vi "build_rid_iterating.vi"(7 "ext":string="_data.h5", 8 "error in (no error)":errorcluster, 9 "save?":bool, 10 "time stamp":timestamp, 11 "base":path[](array[path])) -> (0 "error out":errorcluster, 2 "run ID":string="20180125_155324", 3 "output":path[](array[path]))   [LabVIEW 2017, in "tools.lvlib"]
uses:
  tools.lvlib
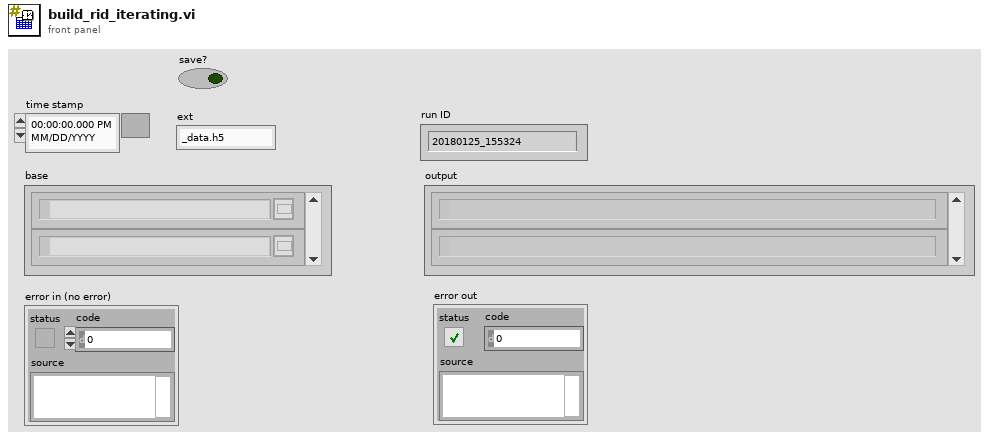
[diagram p1: front panel]
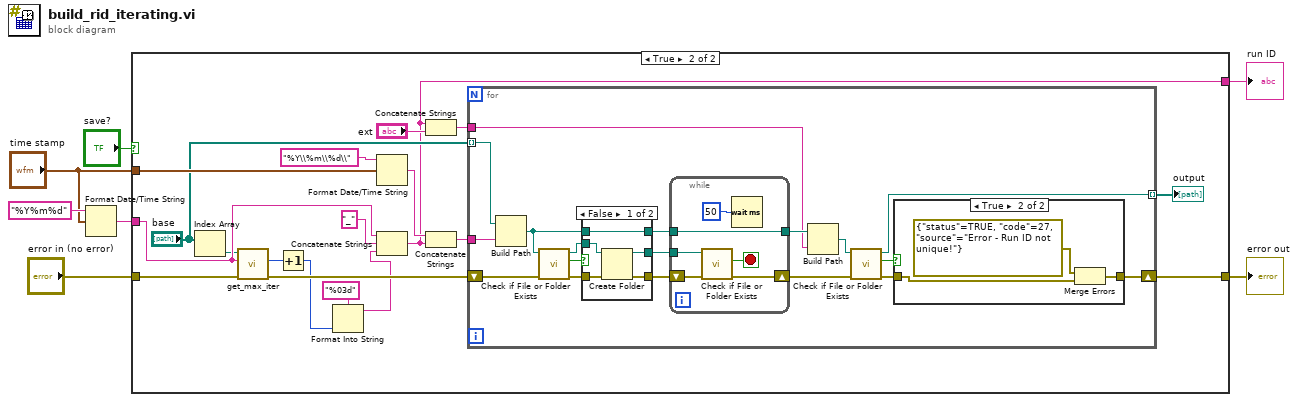
[diagram p0: block diagram]
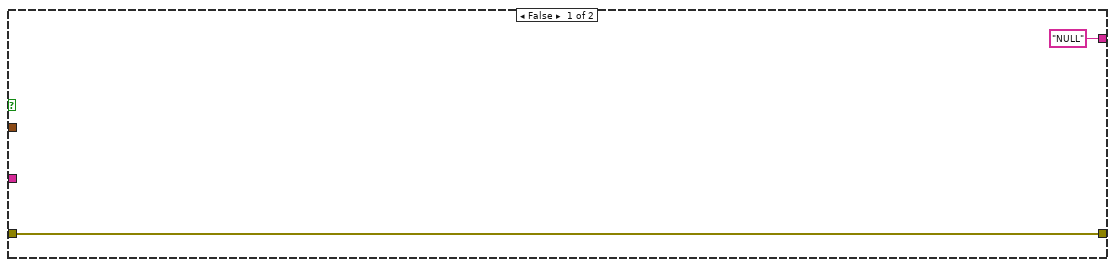
[diagram p2: hidden frame]
diagram:
  n1 = Format Date/Time String(time format string (%c)="%Y%m%d", seconds (now)="time stamp") -> (date/time string=w1:string)  [unwired: 1 in]
  n2 = case shown="True" "save?" {
    tunnel: "time stamp" -> [_ w28]
    tunnel: "error in (no error)" -> [w9 w17]
    tunnel: [w9 w21] -> w3
    tunnel: ["NULL" w13] -> w2
    tunnel: w1 -> [_ w19]
    frame False {
    }
    frame True {
      n3 = Index Array(array="base") -> (element=w14:path)  [unwired: 1 in]
      n4 = call "get_max_iter.vi"("error in"=w17, "date_str"=w19, "base"=w14) -> ("error out"=w16:errorcluster, "max ID"=w18:i32)  [unwired: 3 in, 4 out]
      n5 = Increment(x=w18) -> (x+1=w12:i32)
      n6 = Format Into String(format string="%03d", w12) -> (resulting string=w11:string)  [unwired: 2 in, 1 out]
      n7 = Format Date/Time String(time format string (%c)="%Y\\%m\\%d\\", seconds (now)=w28) -> (date/time string=w26:string)  [unwired: 1 in]
      n8 = Concatenate Strings(w19, "_" ("string"), w11) -> (w13:string)
      n9 = Concatenate Strings(w13, "ext") -> (w23:string)
      n10 = Concatenate Strings(w26, w13) -> (w24:string)
      n11 = for {
        tunnel: "base" -> [w40] mode=indexing
        tunnel: w24 -> [w39]
        tunnel: w23 -> [w38]
        tunnel: [w29] -> w22 mode=indexing
        shift-right: [w31] -> w21
        shift-left: w16 -> [w36]
        n12 = Build Path(base path=w40, name or relative path=w39) -> (appended path=w42:path)
        n13 = call <vilib>:"Check if File or Folder Exists.vi"("error in (no error)"=w36, "path"=w42) -> ("error out"=w37:errorcluster, "file or folder exists?"=w46:bool, "dup path"=w45:path)  [unwired: 7 in]
        n14 = case shown="False" w46 {
          tunnel: w45 -> [w61 w63]
          tunnel: [w60 w64] -> w43
          tunnel: w42 -> [w60 w64]
          tunnel: [w59 w63] -> w44
          tunnel: w37 -> [w58 w62]
          tunnel: [w57 w62] -> w35
          frame False {
            n15 = Create Folder(path (use dialog)=w61, error in=w58) -> (created path=w59:path, error out=w57:errorcluster)  [unwired: 1 in, 1 out]
          }
          frame True {
          }
        }
        n16 = while {
          tunnel: w44 -> [w55]
          tunnel: [w53] -> w41
          tunnel: w43 -> [w53]
          shift-right: [w51] -> w34
          shift-left: w35 -> [w52]
          stop <- w56 stop-if-true
          n17 = call <vilib>:"Check if File or Folder Exists.vi"("error in (no error)"=w52, "path"=w55) -> ("error out"=w51:errorcluster, "file or folder exists?"=w56:bool)  [unwired: 7 in, 1 out]
          n18 = Wait (ms)(milliseconds to wait=u32 50) -> ()  [unwired: 1 out]
        }
        n19 = Build Path(base path=w41, name or relative path=w38) -> (appended path=w30:path)
        n20 = call <vilib>:"Check if File or Folder Exists.vi"("error in (no error)"=w34, "path"=w30) -> ("error out"=w32:errorcluster, "file or folder exists?"=w33:bool, "dup path"=w29:path)  [unwired: 7 in]
        n21 = case shown="True" w33 {
          tunnel: w32 -> [w47 w50]
          tunnel: [w47 w49] -> w31
          frame False {
          }
          frame True {
            n22 = Merge Errors(errorcluster {"status"=TRUE, "code"=27, "source"="Error - Run ID not unique!"} ("error in"), w50) -> (w49:errorcluster)
          }
        }
      }
      "output" <- w22
    }
  }
  "run ID" <- w2
  "error out" <- w3
